vi "To Instrument Session Init and Close Behavior.vi"(10 "session exists":bool, 11 "initialize and close session behavior":T2=enum."Initialize and Close") -> (3 "instrument initialize and close session behavior":T1)   [LabVIEW 2020, in "Measurement Plugin Session Management V1.lvlib" / "Session Reservation.lvclass"]
uses:
  Session Reservation.lvclass
  Initialize and Close Session Behavior.ctl
  MeasurementLink Instrument/ISession Factory/Initialize and Close Session Behavior.ctl
  Session Reservation.lvclass/Session Reservation.ctl
  MeasurementLink Instrument/ISession Factory/ISession Factory.lvclass
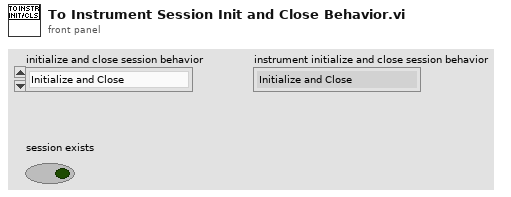
[diagram p1: front panel]
types:
  T1 = typedef "MeasurementLink Instrument.lvlib/ISession Factory.lvclass/Initialize and Close Session Behavior.ctl" = enum16{"Initialize and Close", "Attach and Detach", "Initialize and Detach", "Attach and Close"}
  T2 = typedef "Measurement Plugin Session Management V1.lvlib/Session Reservation.lvclass/Initialize and Close Session Behavior.ctl" = enum16{"Auto", "Initialize and Close", "Attach and Detach", "Initialize and Detach", "Attach and Close"}
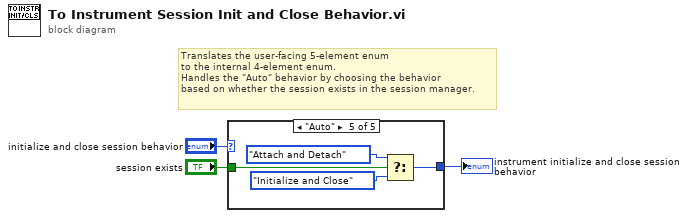
[diagram p0: block diagram]
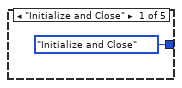
[diagram p2: hidden frame]
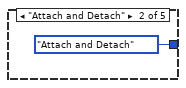
[diagram p3: hidden frame]
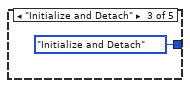
[diagram p4: hidden frame]
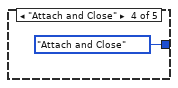
[diagram p5: hidden frame]
diagram:
  # "Translates the user-facing 5-element enum\nto the internal 4-element enum.\nHandles the \"Auto\" behavior by choosing the behavior\nbased on whether the session exists in the session manager."
  n1 = case shown="\"Auto\"" "initialize and close session behavior" {
    tunnel: [Initialize_and_Close_Session_Behavior."Initialize and Close" ("instrument initialize and close session behavior") Initialize_and_Close_Session_Behavior."Attach and Detach" ("instrument initialize and close session behavior") Initialize_and_Close_Session_Behavior."Initialize and Detach" ("instrument initialize and close session behavior") Initialize_and_Close_Session_Behavior."Attach and Close" ("instrument initialize and close session behavior") w8] -> w2
    tunnel: "session exists" -> [_ _ _ _ w11]
    frame "Initialize and Close" {
    }
    frame "Attach and Detach" {
    }
    frame "Initialize and Detach" {
    }
    frame "Attach and Close" {
    }
    frame "Auto" {
      n2 = Select(t=Initialize_and_Close_Session_Behavior."Attach and Detach" ("instrument initialize and close session behavior"), s=w11, f=Initialize_and_Close_Session_Behavior."Initialize and Close") -> (s? t:f=w8:T1)
    }
  }
  "instrument initialize and close session behavior" <- w2
